vi "send_radar_cube_flag.vi"(4 "error in":errorcluster, 7 "Radar configuration":string="{\n  \"type\": \"Radar\",\n   \"gpu_number\":0,\n  \"listen_port\": 8301,\n  \"send_radar_cube\":false,\n  \"paint_targets\": false,\n  \"target_paint_lifetime\": 0.5,\n  \"location\": {\n    \"x\": 250.0,\n    \"y\": 0.0,\n    \"z\": 50.0\n  },\n  \"rotation\": {\n    \"pitch\": 0.0,\n    \"yaw\": 0.0,\n    \"roll\": 0.0\n  },\n  \"num_samples_per_sweep\":345,\n  \"fs\": 50000000,\n  \"fc\": 77000000000.0,\n  \"num_sweeps\": 32,\n  \"sweep_time\" : 0.0000069,\n  \"bandwidth\" : 172500000,\n  \"max_targets\": 250,\n  \"elements\": 8,\n  \"transmitter\": {\n    \"peak_power\": 5.0,\n    \"aperture\": 0.000859,\n    \"gain\": 13.50\n  },\n  \"receiver\": {\n    \"aperture\": 0.000798,\n    \"nf\": 10.0,\n    \"noise_temp\": 290.0,\n    \"nb\": 74000000.0,\n    \"gain\": 10.0\n  },\n  \"sbr\": {\n    \"long_range_scan_distance\": 150.0,\n    \"short_range_scan_distance\": 60.0,\n    \"long_range_fov\": 20.0,\n    \"short_range_fov\": 60.0,\n    \"elevation_fov\": 10.0,\n    \"rescan_density\": 20.0,\n    \"debug_frustum\": false,\n    \"debug_scan\": false,\n    \"debug_rescan\": false\n  }\n}") -> (0 "error out":errorcluster, 3 "send_radar_cube":bool)   [LabVIEW 2019]
doc: "Check if the flag *send_radar_cube* is available on the configuration."
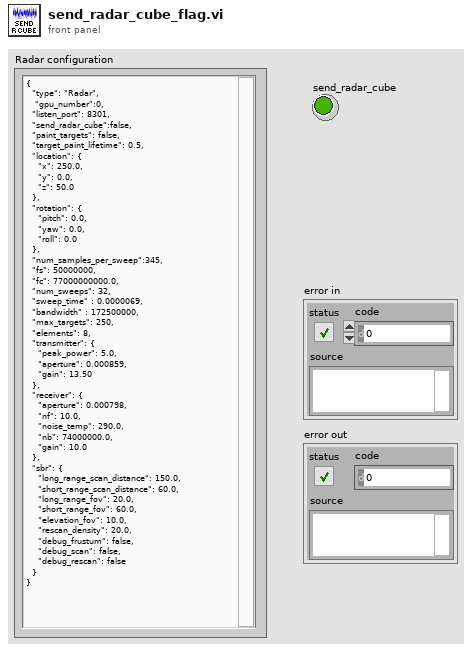
[diagram p1: front panel]
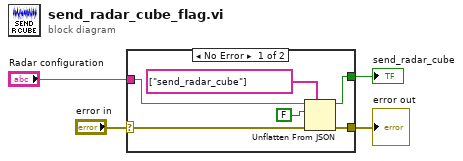
[diagram p0: block diagram]
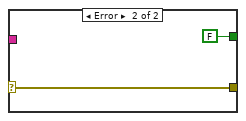
[diagram p2: hidden frame]
diagram:
  n1 = case shown="No Error" "error in" {
    selector: "error in" -> [w8 w12]
    tunnel: "Radar configuration" -> [w7 _]
    tunnel: [w5 FALSE ("f")] -> w3
    tunnel: [w6 w12] -> w2
    frame No Error {
      n2 = Unflatten From JSON(path=string[] ["send_radar_cube"], JSON string=w7, type and defaults=FALSE, error in (no error)=w8) -> (value=w5:bool, error out=w6:errorcluster)  [unwired: 3 in]
    }
    frame Error {
    }
  }
  "send_radar_cube" <- w3
  "error out" <- w2
